vi "Radar2_rev1.vi"() -> ()   [LabVIEW 2018]
panel:
  in  "Angle":dbl(slide)=60.0 min=0.0 max=360.0 step=10.0 scale=0.0..360.0
  in  "Distance":dbl(slide)=60.0 min=0.0 max=100.0 step=1.0 scale=0.0..100.0
  out "ping":bool
  in  "stop":bool
  out "2D Picture":picture
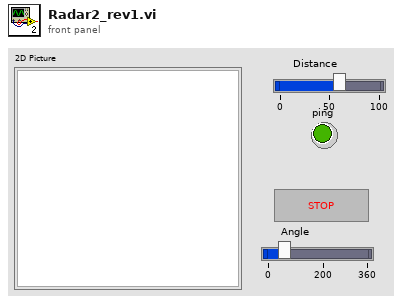
[diagram p1: front panel]
types:
  T1 = cluster{"maximum":dbl, "minimum":dbl, "clip to min":bool, "log?(F)":bool, "grid color":u32, "plot color":u32, "fmt and prec":cluster{"format":enum8{"Decimal", "Scientific", "Engineering", "Binary", "Octal", "Hex"}, "precision":u8}, "visible section":u16}
  T2 = cluster{"Width":u16, "Style":enum32{"Solid", "Dash", "Dot", "DashDot", "DashDotDot"}}
  T3 = typedef "imagedata.ctl" = cluster{"image type":i32, "image depth":i32, "image":u8[], "mask":u8[], "colors":u32[], "Rectangle":cluster{"left":i16, "top":i16, "right":i16, "bottom":i16}}
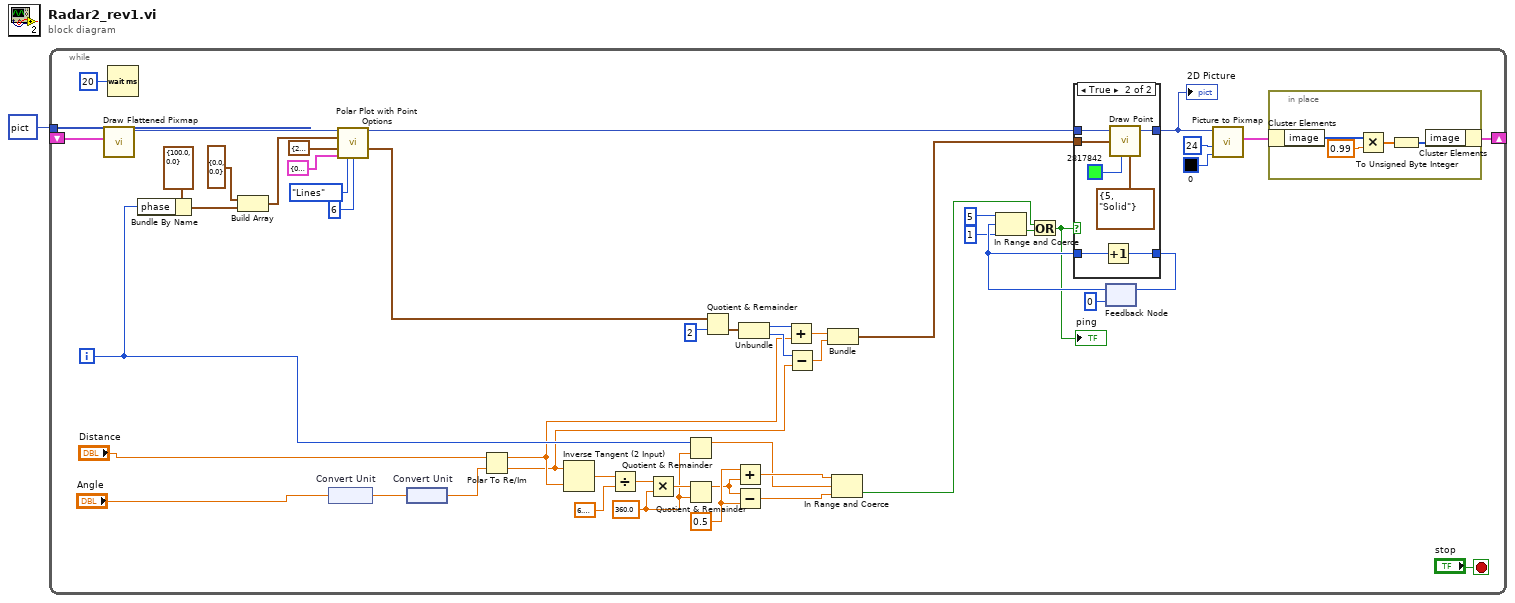
[diagram p0: block diagram]
diagram:
  n1 = while {
    shift-right: [w47] -> _
    shift-left: _ -> [w46]
    tunnel: picture data[5B] ("2D Picture") -> [w45]
    i -> [w24]
    stop <- "stop" stop-if-true
    w22 = 0.5
    w15 = 360.0 ("y")
    w35 = cluster{"width":i16, "height":i16} {"width"=222, "height"=222} ("dimensions (w,h)")
    n2 = call <vilib>:"Draw Flattened Pixmap.vi"("image data"=w46, "picture"=w45) -> ("new picture"=w52:picture)  [unwired: 7 in]
    n3 = Wait (ms)(milliseconds to wait=u32 20) -> ()  [unwired: 1 out]
    n4 = Bundle By Name(cluster=cluster{"magnitude":dbl, "phase":dbl} {"magnitude"=100.0, "phase"=0.0}, "phase"=w24) -> (w43:cluster{"magnitude":dbl, "phase":dbl})
    n5 = Build Array(cluster{"magnitude":dbl, "phase":dbl} {"magnitude"=0.0, "phase"=0.0}, w43) -> (w39:cluster{"magnitude":dbl, "phase":dbl}[])
    n6 = node "Convert Unit"("Angle") -> (w4:dbl[unit])
    n7 = call <vilib>:"Polar Plot with Point Options.vi"("picture"=w52, "data array [mag, phase (deg)]"=w39, "dimensions (w,h)"=w35, "polar attributes"=T1 {"maximum"=0.0, "minimum"=0.0, "clip to min"=FALSE, "log?(F)"=FALSE, "grid color"=6710886, "plot color"=2465536, "fmt and prec"={"format"=enum."Decimal", "precision"=0}, "visible section"=8}, "Lines/Points"=enum16{"Lines", "Points"}."Lines", "Size"=u16 6) -> ("new picture"=w51:picture)  [unwired: 9 in]
    n8 = node "Convert Unit"(w4) -> (w5:dbl)
    n9 = Polar To Re/Im(2:w5, 3:"Distance") -> (0:w6:dbl, 1:w7:dbl)
    n10 = Inverse Tangent (2 Input)(1:w7, 2:w6) -> (0:w19:dbl)
    n11 = Divide(x=w19, y=6.283185307179586) -> (x/y=w18:dbl)
    n12 = Multiply(x=w18, y=w15) -> (x*y=w17:dbl)
    n13 = Quotient & Remainder(x=w24, y=w15) -> (x-y*floor(x/y)=w14:dbl)  [unwired: 1 out]
    n14 = Quotient & Remainder(x=w17, y=w15) -> (x-y*floor(x/y)=w16:dbl)  [unwired: 1 out]
    n15 = Quotient & Remainder(x=w35, y=i16 2) -> (floor(x/y)=w12:cluster{"width":i16, "height":i16})  [unwired: 1 out]
    n16 = Add(x=w22, y=w16) -> (x+y=w21:dbl)
    n17 = Subtract(x=w16, y=w22) -> (x-y=w20:dbl)
    n18 = Unbundle(w12) -> ("width"=w11:i16, "height"=w10:i16)
    n19 = Add(x=w11, y=w7) -> (x+y=w9:dbl)
    n20 = Subtract(x=w10, y=w6) -> (x-y=w8:dbl)
    n21 = Bundle(w9, w8) -> (w34:cluster{dbl, dbl})  [unwired: 1 in]
    n22 = In Range and Coerce(upper limit=w21, x=w14, lower limit=w20) -> (In Range?=w29:bool)  [unwired: 1 out]
    n23 = feedback #1(u8 0) -> (w28:u8)
    n24 = In Range and Coerce(upper limit=u8 5 ("y"), x=w28, lower limit=u8 1) -> (In Range?=w30:bool)  [unwired: 1 out]
    n25 = Or(x=w29, y=w30) -> (x .or. y?=w25:bool)
    "ping" <- w25
    n26 = case shown="True" w25 {
      tunnel: w51 -> [w53 w60]
      tunnel: [w53 w59] -> w37
      tunnel: w34 -> [_ w58]
      tunnel: [_ w55] -> w32
      tunnel: w28 -> [_ w54]
      frame False {
      }
      frame True {
        n27 = Increment(x=w54) -> (x+1=w55:u8)
        n28 = call <vilib>:"Draw Point.vi"("picture"=w60, "point(x,y)"=w58, "color(black)"=u32 2817842 ("plot color"), "pen"=T2 {"Width"=5, "Style"=enum."Solid"}) -> ("new picture"=w59:picture)  [unwired: 5 in]
      }
    }
    "2D Picture" <- w37
    n29 = feedback-in #1(w32) -> ()
    n30 = call <vilib>:"Picture to Pixmap.vi"("Background Color"=u32 0, "depth"=24, "picture"=w37) -> ("image data"=w48:T3)  [unwired: 7 in, 1 out]
    n31 = in-place {
      n32 = in-place-cluster #2(w48) -> ("image"=w64:u8[])
      n33 = Multiply(x=w64, y=0.99) -> (x*y=w62:dbl[])
      n34 = To Unsigned Byte Integer(number=w62) -> (unsigned 8bit integer=w61:u8[])
      n35 = in-place-cluster #2("image"=w61) -> (w47:T3)
    }
  }
